vi "do_determine_c_parameter.vi"   [LabVIEW 2019]
types:
  T1 = typedef "xi_angles_enum_typedef.ctl" = enum16{"0", "45"}
  T2 = cluster{"Global Rectangle":i32[], "Contours":cluster{"Contour Type":u32, "ROI Type":u32, "Points":i32[]}[]}
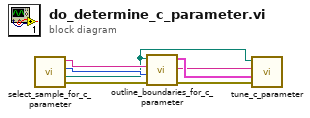
[diagram p0: block diagram]
diagram:
  n1 = call "select_sample_for_c_parameter.vi"() -> ("Error Out"=w5:errorcluster, "selected path"=w4:path, "Xi"=w6:T1, "Selected Sample"=w7:string)  [unwired: 8 in]
  n2 = call "outline_boundaries_for_c_parameter.vi"("Error In"=w5, "Xi"=w6, "Sample"=w7, "File Path"=w4) -> ("Error Out"=w1:errorcluster, "Image"=w2:string, "ROI"=w3:T2)  [unwired: 5 in]
  n3 = call "tune_c_parameter.vi"("Error In"=w1, "ROI"=w3, "original image name"=w2, "File Path"=w4) -> ()  [unwired: 7 in, 1 out]
